vi "Table Section.vi"(8 "error in (no error)":errorcluster, 11 "Node Ptr":T1 format="%.0x") -> (0 "error out":errorcluster)   [LabVIEW 2020, in "Profile Interpolation System Explorer.lvlib"]
uses:
  Profile Interpolation System Explorer.lvlib
  <vilib>/NI VeriStand/Custom Device API/Custom Device Item Ref.ctl
  Shared/Types/FG Action.ctl
  <vilib>/NI VeriStand/Custom Device Tools/Custom Device Utility Library/Search Direction.ctl
  <vilib>/Utility/miscctls.llb/LVRowAndColumnTypeDef.ctl
  Shared/SubVIs/Constants.vi
  <vilib>/NI VeriStand/Custom Device Tools/Custom Device Utility Library/NI VeriStand - Search for Item by GUID.vi
  <vilib>/NI VeriStand/Custom Device API/NI VeriStand - Get Item Property.vi
  <vilib>/NI VeriStand/Custom Device API/Get Item Property (Path).vi
  <vilib>/NI VeriStand/Custom Device API/Get Item Property (Boolean).vi
  <vilib>/NI VeriStand/Custom Device API/NI VeriStand - Set Item Property.vi
  <vilib>/NI VeriStand/Custom Device API/Set Item Property (Path).vi
  <vilib>/NI VeriStand/Custom Device API/Set Item Property (Boolean).vi
  <vilib>/NI VeriStand/Custom Device API/Custom Device API.lvlib
  Shared/Profile Interpolation Shared.lvlib
  <vilib>/NI VeriStand/Custom Device Tools/Custom Device Utility Library/Custom Device Utility Library.lvlib
panel:
  out "Table":string[][](table)
  in  "SHDocVw.IWebBrowser":refnum<k7>(container)
  in  "Specific Header":cluster{"Section Name":string}={"Section Name"="Specific Page Settings"}
  in  "General Header":cluster{"Section Name":string}={"Section Name"="General Page Settings"}
  in  "Description":string
  in  "Name":string
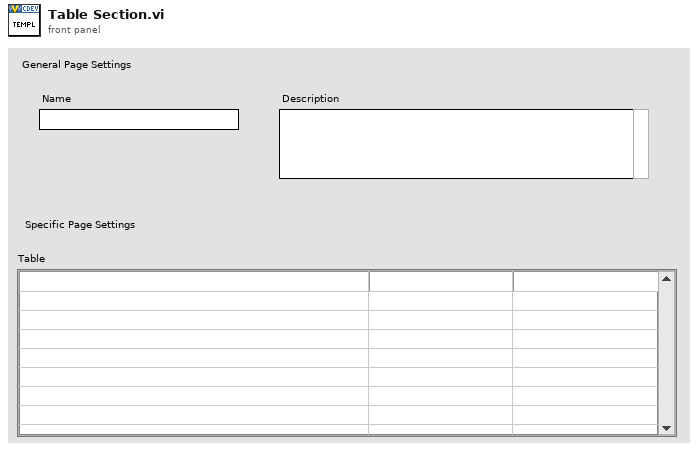
[diagram p1: front panel]
types:
  T1 = typedef "Custom Device API.lvlib/Custom Device Item Ref.ctl" = u64
  T2 = typedef "Custom Device Utility Library.lvlib/Search Direction.ctl" = enum16{"Down", "Up"}
  T3 = typedef "Profile Interpolation Shared.lvlib/FG Action.ctl" = enum8{"GET", "SET"}
  T4 = typedef "LVRowAndColumnTypeDef.ctl" = cluster{"Row":i32, "Column":i32}
  T5 = typedef "Profile Interpolation Shared.lvlib/Interpolation Settings.ctl" = cluster{"Interpolation File":path, "Create Limit Channels?":bool}
  T6 = typedef "Custom Device API.lvlib/Custom Device Item Info.ctl" = cluster{"Name":string, "Is Channel":bool, "GUID":string, "Is Waveform":bool}
  T7 = typedef "Custom Device API.lvlib/Custom Device Commands.ctl" = enum16{"Default", "Item renamed", "Shutdown", "Dynamic button pressed"}
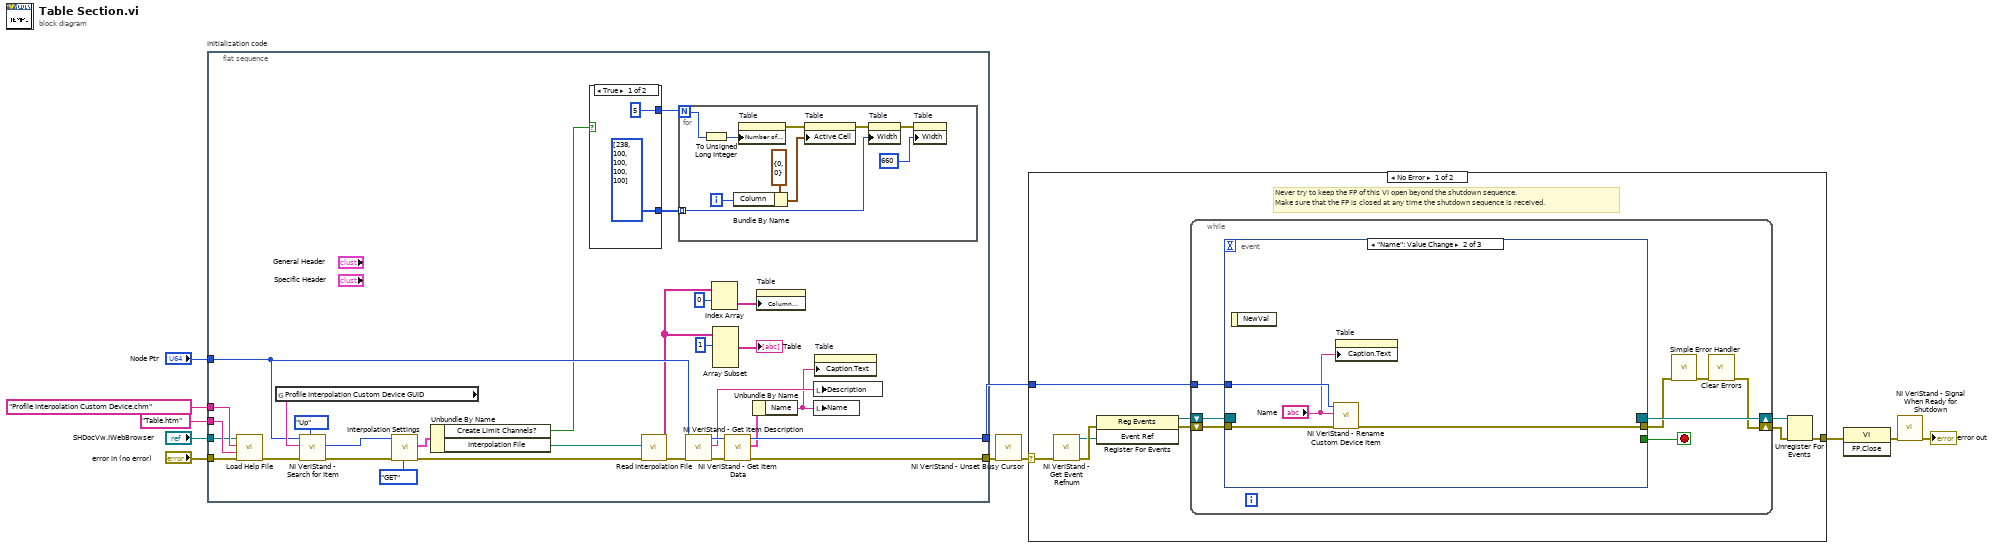
[diagram p0: block diagram]
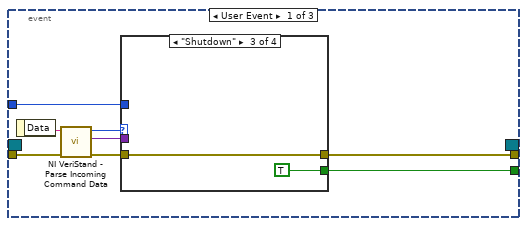
[diagram p2: hidden frame]
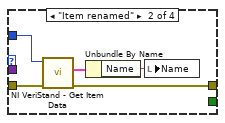
[diagram p4: hidden frame]
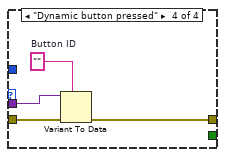
[diagram p5: hidden frame]
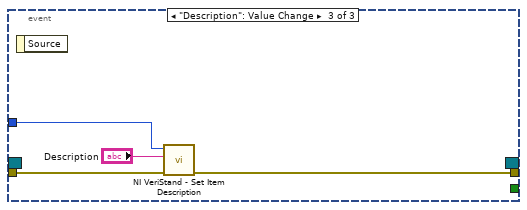
[diagram p6: hidden frame]
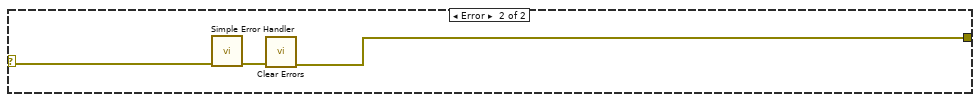
[diagram p7: hidden frame]
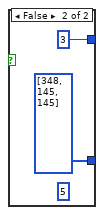
[diagram p8: hidden frame]
diagram:
  n1 = flat-sequence "Initialization code" {
    tunnel: "error in (no error)" -> [w36]
    tunnel: "Node Ptr" -> [w23]
    tunnel: [w37] -> w7
    tunnel: [w41] -> w4
    tunnel: "SHDocVw.IWebBrowser" -> [w33]
    tunnel: "Table.htm" ("CD_CHM_Section") -> [w35]
    tunnel: "Profile Interpolation Custom Device.chm" ("CD_CHM_FileName") -> [w34]
    frame #0 {
      n2 = call "Load Help File.vi"("error in (no error)"=w36, "HTML File"=w35, "Main CHM File"=w34, "SHDocVw.IWebBrowser2"=w33) -> ("error out"=w25:errorcluster)  [unwired: 7 in]
      n3 = global read "Constants.vi" "Profile Interpolation Custom Device GUID"() -> (w30:string)
      n4 = call-poly <vilib>:"NI VeriStand - Search for Item.vi"("Direction (Down)"=Search_Direction."Up", "error in"=w25, "Item GUID"=w30, "Section Ref in"=w23) -> ("error out"=w31:errorcluster, "Item Ref"=w17:T1)  [unwired: 4 in, 2 out]
      n5 = call "Interpolation Settings.vi"("Action"=FG_Action."GET", "error in (no error)"=w31, "Item Ref"=w17) -> ("error out"=w28:errorcluster, "Interpolation Settings out"=w15:T5)  [unwired: 6 in, 1 out]
      n6 = Unbundle By Name(w15) -> ("Create Limit Channels?"=w12:bool, "Interpolation File"=w29:path)
      n7 = case shown="True" w12 {
        tunnel: [5 ("f") 3 ("f")] -> w13
        tunnel: [u32[] [238, 100, 100, 100, 100] u32[] [348, 145, 145]] -> w14
        frame True {
        }
        frame False {
          (unwired) 5 ("f")
        }
      }
      n8 = call "Read Interpolation File.vi"("error in"=w28, "file path (dialog if empty)"=w29) -> ("error out"=w24:errorcluster, "Raw Data"=w20:string[][])  [unwired: 2 in, 6 out]
      n9 = for {
        N: w13 -> [w46]
        tunnel: w14 -> [w44] mode=indexing
        i -> [w50]
        n10 = To Unsigned Long Integer(number=w46) -> (unsigned 32bit integer=w45:u32)
        n11 = Bundle By Name(cluster=T4 {"Row"=0, "Column"=0} ("Active Cell:Active Cell"), "Column"=w50) -> (w51:T4)
        n12 = property on="Table" class="Tbl (strict)"("Number of Columns"=w45) -> (error out=w47:errorcluster)  [unwired: 2 in, 1 out]
        n13 = property on="Table" class="Tbl (strict)"(error in=w47, "Active Cell"=w51) -> (error out=w49:errorcluster)  [unwired: 1 in, 1 out]
        n14 = property on="Table" class="Tbl (strict)"(error in=w49, "Width"=w44) -> (error out=w43:errorcluster)  [unwired: 1 in, 1 out]
        n15 = property on="Table" class="Tbl (strict)"(error in=w43, "Width"=u32 660 ("Size:Width")) -> ()  [unwired: 1 in, 2 out]
      }
      n16 = call <vilib>:"NI VeriStand - Get Item Description.vi"("error in (no error)"=w24, "Item Ref in"=w23) -> ("error out"=w39:errorcluster, "Description"=w32:string, "Item Ref out"=w40:T1)  [unwired: 7 out]
      n17 = Index Array(array=w20, index (row)=0) -> (element=w21:string[])  [unwired: 1 in]
      n18 = Array Subset(array=w20, index (row)=1 ("index")) -> (→"Table":string[][])  [unwired: 3 in]
      n19 = call <vilib>:"NI VeriStand - Get Item Data.vi"("error in (no error)"=w39, "Item Ref in"=w40) -> ("error out"=w37:errorcluster, "Item Info"=w38:T6, "Item Ref out"=w41:T1)  [unwired: 7 out]
      n20 = Unbundle By Name(w38) -> ("Name"=w16:string)
      n21 = property on="Table" class="Tbl (strict)"("Column Headers[]"=w21) -> ()  [unwired: 2 in, 2 out]
      n22 = local write "Description"(w32) -> ()
      n23 = local write "Name"(w16) -> ()
      n24 = property on="Table" class="Tbl (strict)"("Caption.Text"=w16) -> ()  [unwired: 2 in, 2 out]
    }
  }
  n25 = call <vilib>:"NI VeriStand - Unset Busy Cursor.vi"("error in (no error)"=w7) -> ("error out"=w6:errorcluster)  [unwired: 10 out]
  n26 = case shown="No Error" w6 {
    selector: w6 -> [w56 w103]
    tunnel: [w61 w101] -> w11
    tunnel: w4 -> [w57 _]
    frame No Error {
      # "Never try to keep the FP of this VI open beyond the shutdown sequence.\nMake sure that the FP is closed at any time the shutdown sequence is received."
      n27 = call <vilib>:"NI VeriStand - Get Event Refnum.vi"("error in (no error)"=w56) -> ("error out"=w64:errorcluster, "Event Ref"=w60:refnum<user-event>)  [unwired: 9 out]
      n28 = register-events(error in=w64, w60) -> (reference out=w58:refnum<event-registration>, error out=w59:errorcluster)  [unwired: 1 in]
      n29 = while {
        tunnel: w57 -> [w68]
        shift-right: [w65] -> w62
        shift-left: w59 -> [w71]
        shift-right: [w72] -> w63
        shift-left: w58 -> [w70]
        stop <- w69 stop-if-true
        n30 = event shown="[1] \"Name\": Value Change" {
          selector: w70 -> [_ _ _]
          dyn-events: [_ _ _] -> w72
          timeout: _ -> [_ _ _]
          tunnel: w71 -> [w80 w96 w99]
          tunnel: [w76 _ _] -> w69
          tunnel: [w75 w95 w98] -> w67
          tunnel: w68 -> [w74 w94 w100]
          event User Event {
            n31 = event-data() -> ("Data"=w79:string)  [unwired: 1 out]
            n32 = call <vilib>:"NI VeriStand - Parse Incoming Command Data.vi"("error in (no error)"=w80, "Incoming data"=w79) -> ("error out"=w78:errorcluster, "Outgoing data"=w73:variant, "Action"=w77:T7)  [unwired: 7 out]
            n33 = case shown="\"Shutdown\"" w77 {
              tunnel: w78 -> [w81 w86 w87 w92]
              tunnel: [_ _ TRUE _] -> w76
              tunnel: [w81 w83 w87 w89] -> w75
              tunnel: w74 -> [_ w85 _ _]
              tunnel: w73 -> [_ _ _ w91]
              frame "Default", Default {
              }
              frame "Item renamed" {
                n34 = call <vilib>:"NI VeriStand - Get Item Data.vi"("error in (no error)"=w86, "Item Ref in"=w85) -> ("error out"=w83:errorcluster, "Item Info"=w84:T6)  [unwired: 8 out]
                n35 = Unbundle By Name(w84) -> ("Name"=w82:string)
                n36 = local write "Name"(w82) -> ()
              }
              frame "Shutdown" {
              }
              frame "Dynamic button pressed" {
                w90 = ""  # Button ID
                n37 = Variant To Data(error in=w92, type=w90, Variant=w91) -> (error out=w89:errorcluster)  [unwired: 1 out]
              }
            }
          }
          event "Name": Value Change {
            n38 = event-data() -> ()  [unwired: 2 out]
            n39 = call <vilib>:"NI VeriStand - Rename Custom Device Item.vi"("error in (no error)"=w96, "New Name"="Name", "Item Ref in"=w94) -> ("error out"=w95:errorcluster)  [unwired: 1 in, 7 out]
            n40 = property on="Table" class="Tbl (strict)"("Caption.Text"="Name") -> ()  [unwired: 2 in, 2 out]
          }
          event "Description": Value Change {
            n41 = event-data() -> ()  [unwired: 2 out]
            n42 = call <vilib>:"NI VeriStand - Set Item Description.vi"("error in (no error)"=w99, "Description"="Description", "Item Ref in"=w100) -> ("error out"=w98:errorcluster)  [unwired: 8 out]
          }
        }
        n43 = call <vilib>:"Simple Error Handler.vi"("error in (no error)"=w67) -> ("error out"=w66:errorcluster)  [unwired: 1 in, 7 out]
        n44 = call <vilib>:"Clear Errors.vi"("error in (no error)"=w66) -> ("error out"=w65:errorcluster)  [unwired: 1 in, 5 out]
      }
      n45 = Unregister For Events(event registration refnum=w63, error in=w62) -> (error out=w61:errorcluster)
    }
    frame Error {
      n46 = call <vilib>:"Simple Error Handler.vi"("error in (no error)"=w103) -> ("error out"=w102:errorcluster)  [unwired: 1 in, 7 out]
      n47 = call <vilib>:"Clear Errors.vi"("error in (no error)"=w102) -> ("error out"=w101:errorcluster)  [unwired: 1 in, 5 out]
    }
  }
  n48 = invoke class="VI" method="FP.Close"(error in=w11) -> (error out=w10:errorcluster)  [unwired: 2 in, 2 out]
  n49 = call <vilib>:"NI VeriStand - Signal When Ready for Shutdown.vi"("error in (no error)"=w10) -> ("error out"=→"error out":errorcluster)  [unwired: 10 out]
